vi "Reset.vi"(8 "error in (no error)":errorcluster, 11 "PCA in":refnum<class "PCA.lvclass">) -> (0 "error out":errorcluster, 3 "PCA out":refnum<class "PCA.lvclass">)   [LabVIEW 2022 SP3, in "PCA9685.lvlib" / "PCA.lvclass"]
uses:
  PCA.lvclass
  PCA.lvclass/PCA.ctl
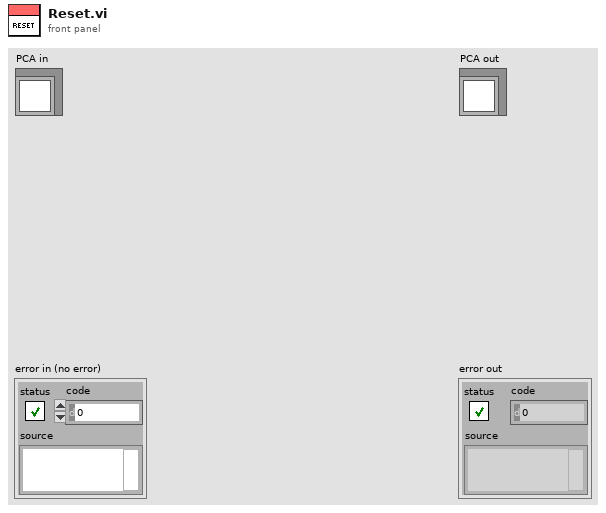
[diagram p1: front panel]
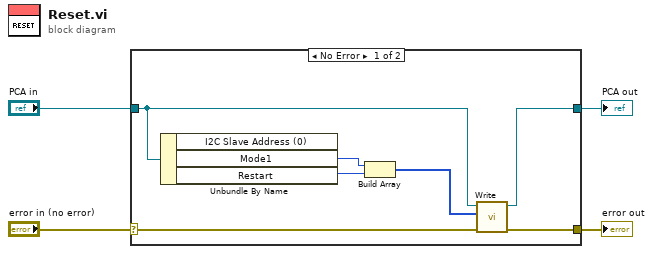
[diagram p0: block diagram]
diagram:
  n1 = case shown="No Error" "error in (no error)" {
    selector: "error in (no error)" -> [w9 w13]
    tunnel: [w8 w13] -> w3
    tunnel: [w6 w12] -> w1
    tunnel: "PCA in" -> [w7 w12]
    frame No Error {
      n2 = Unbundle By Name(w7) -> ("Mode1"=w11:u8, "Restart"=w10:u8)  [unwired: 1 out]
      n3 = Build Array(w11, w10) -> (w5:u8[])
      n4 = call "Write.vi"("error in (no error)"=w9, "Data"=w5, "PCA in"=w7) -> ("error out"=w8:errorcluster, "PCA out"=w6:refnum<class "PCA.lvclass">)  [unwired: 7 in]
    }
    frame Error {
    }
  }
  "error out" <- w3
  "PCA out" <- w1
